vi "Pneumatics_Execute.vi"(8 "error in":errorcluster, 11 "Robot Mode":T1) -> (0 "error out":errorcluster)   [LabVIEW 2020]
uses:
  <vilib>/Rock Robotics/WPI/DriverStation/WPI_DriverStationRobotMode2.ctl
  <vilib>/Rock Robotics/WPI/Solenoid/WPI_SolenoidValue.ctl
  <vilib>/Rock Robotics/Network Tables/NT Write Boolean.vi
  <vilib>/Rock Robotics/Network Tables/NT Write Integer.vi
  <vilib>/Rock Robotics/WPI/Solenoid/WPI_SolenoidSetEnum.vi
  <vilib>/Rock Robotics/Network Tables/NT Read Boolean.vi
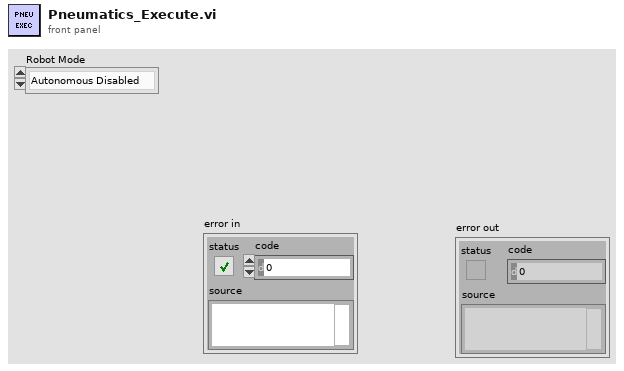
[diagram p1: front panel]
types:
  T1 = typedef "WPI_DriverStationRobotMode2.ctl" = enum16{"Autonomous Disabled", "Autonomous Enabled", "Teleop Disabled", "Teleop Enabled", "Disconnected", "Finish", "Test Disabled", "Test Enabled", "Emergency Stopped"}
  T2 = typedef "WPI_SolenoidValue.ctl" = enum16{"Off", "On", "Forward", "Reverse"}
  T3 = typedef "WPI_SwitchDevRef.ctl" = cluster{"DevStatus":errorcluster, "DIO Channel":T4, "CntIndex":T5, "Normally Closed":bool}
  T4 = typedef "FPGA_DIOChannel.ctl" = enum8{"DIO 0", "DIO 1", "DIO 2", "DIO 3", "DIO 4", "DIO 5", "DIO 6", "DIO 7", "DIO 8", "DIO 9", "DIO MXP 0", "DIO MXP 1", "DIO MXP 2", "DIO MXP 3", "DIO MXP 4", "DIO MXP 5", "DIO MXP 6", "DIO MXP 7", "DIO MXP 8", "DIO MXP 9", "DIO MXP 10", "DIO MXP 11", "DIO MXP 12", "DIO MXP 13", "DIO MXP 14", "DIO MXP 15", "SPI Port CS1", "SPI Port CS2", "SPI Port CS3", "SPI Port MISO", "SPI Port MOSI", "Invalid"}
  T5 = typedef "FPGA_CounterCtrSystemIndex.ctl" = enum8{"Ctr 0", "Ctr 1", "Ctr 2", "Ctr 3", "Ctr 4", "Ctr 5", "Ctr 6", "Ctr 7", "Invalid"}
  T6 = typedef "WPI_SolenoidDevRef.ctl" = cluster{"DevStatus":errorcluster, "Pneumatics Control Module":u8, "Forward Solenoid Channel":T7, "Reverse Solenoid Channel":T7}
  T7 = typedef "WPI_SolenoidChannel.ctl" = enum8{"Solenoid 0", "Solenoid 1", "Solenoid 2", "Solenoid 3", "Solenoid 4", "Solenoid 5", "Solenoid 6", "Solenoid 7", "Solenoid 8", "Solenoid 9", "Solenoid 10", "Solenoid 11", "Solenoid 12", "Solenoid 13", "Solenoid 14", "Solenoid 15", "Invalid"}
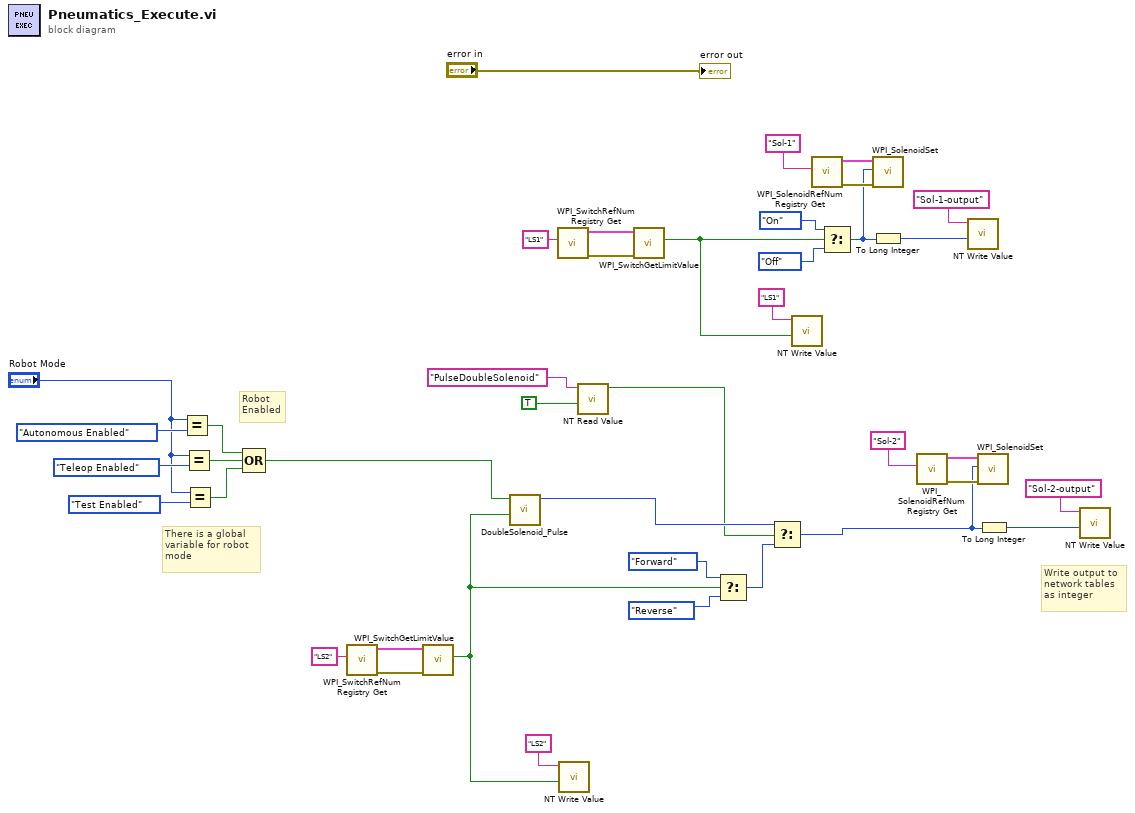
[diagram p0: block diagram]
diagram:
  # "Robot\nEnabled"
  # "There is a global \nvariable for robot \nmode"
  # "Write output to\nnetwork tables\nas integer"
  n1 = Equal?(x="Robot Mode", y=WPI_DriverStationRobotMode2."Autonomous Enabled") -> (x = y?=w22:bool)
  n2 = Equal?(x="Robot Mode", y=WPI_DriverStationRobotMode2."Teleop Enabled") -> (x = y?=w21:bool)
  n3 = Equal?(x="Robot Mode", y=WPI_DriverStationRobotMode2."Test Enabled") -> (x = y?=w20:bool)
  n4 = Compound Arithmetic op=OR(w22, w21, w20) -> (w19:bool)
  n5 = call <vilib>:"WPI_SwitchRefNum Registry Get.vi"("refnum name"="LS2") -> ("error out"=w12:errorcluster, "SwitchDevRef"=w13:T3)  [unwired: 9 in]
  n6 = call <vilib>:"WPI_SwitchGetLimitValue.vi"("error in (no error)"=w12, "SwitchDevRef"=w13) -> ("Switch Pressed"=w4:bool)  [unwired: 7 in, 2 out]
  n7 = call "DoubleSolenoid_Pulse.vi"("Solenoid Demand"=w4, "Robot Enabled"=w19) -> ("Solenoid Cmd"=w6:T2)  [unwired: 9 in]
  n8 = call <vilib>:"WPI_SwitchRefNum Registry Get.vi"("refnum name"="LS1") -> ("error out"=w17:errorcluster, "SwitchDevRef"=w18:T3)  [unwired: 9 in]
  n9 = call-poly <vilib>:"NT Write Value.vi"("value"=w4, "name"="LS2") -> ()  [unwired: 9 in, 1 out]
  n10 = call-poly <vilib>:"NT Read Value.vi"("default value"=TRUE, "name"="PulseDoubleSolenoid") -> ("value"=w1:bool)  [unwired: 7 in, 2 out]
  n11 = call <vilib>:"WPI_SwitchGetLimitValue.vi"("error in (no error)"=w17, "SwitchDevRef"=w18) -> ("Switch Pressed"=w14:bool)  [unwired: 7 in, 2 out]
  n12 = Select(t=WPI_SolenoidValue."Forward" ("Solenoid Cmd"), s=w4, f=WPI_SolenoidValue."Reverse" ("Solenoid Cmd")) -> (s? t:f=w5:T2)
  n13 = Select(t=w6, s=w1, f=w5) -> (s? t:f=w3:T2)
  n14 = call-poly <vilib>:"NT Write Value.vi"("value"=w14, "name"="LS1") -> ()  [unwired: 9 in, 1 out]
  n15 = call <vilib>:"WPI_SolenoidRefNum Registry Get.vi"("refnum name"="Sol-1") -> ("error out"=w38:errorcluster, "SolenoidDevRef"=w37:T6)  [unwired: 9 in]
  n16 = Select(t=WPI_SolenoidValue."On" ("Value"), s=w14, f=WPI_SolenoidValue."Off" ("Value")) -> (s? t:f=w31:T2)
  n17 = call-poly <vilib>:"WPI_SolenoidSet.vi"("error in (no error)"=w38, "Value"=w31, "SolenoidDevRef"=w37) -> ()  [unwired: 7 in, 2 out]
  n18 = To Long Integer(number=w31) -> (32bit integer=w27:i32)
  n19 = call <vilib>:"WPI_SolenoidRefNum Registry Get.vi"("refnum name"="Sol-2") -> ("error out"=w33:errorcluster, "SolenoidDevRef"=w32:T6)  [unwired: 9 in]
  n20 = call-poly <vilib>:"NT Write Value.vi"("value"=w27, "name"="Sol-1-output") -> ()  [unwired: 9 in, 1 out]
  n21 = call-poly <vilib>:"WPI_SolenoidSet.vi"("error in (no error)"=w33, "Value"=w3, "SolenoidDevRef"=w32) -> ()  [unwired: 7 in, 2 out]
  n22 = To Long Integer(number=w3) -> (32bit integer=w29:i32)
  n23 = call-poly <vilib>:"NT Write Value.vi"("value"=w29, "name"="Sol-2-output") -> ()  [unwired: 9 in, 1 out]
  "error out" <- "error in"
